vi "Self-Test.vi"(7 "Address":u16, 8 "Error In":errorcluster, 11 "VISA Resource in":refnum<visa-resource-name>) -> (0 "Error Out":errorcluster, 1 "Self-Test Result Message":string, 2 "Self-Test Result Code":i32, 3 "VISA Resource out":refnum<visa-resource-name>)   [LabVIEW 2014, in "KIT QV.lvlib"]
doc: "Runs the instrument's self-test routine and returns the test results."
uses:
  KIT QV.lvlib
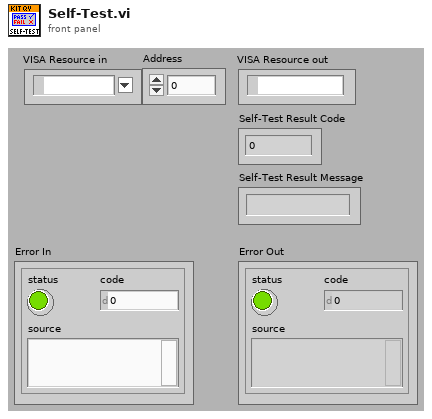
[diagram p1: front panel]
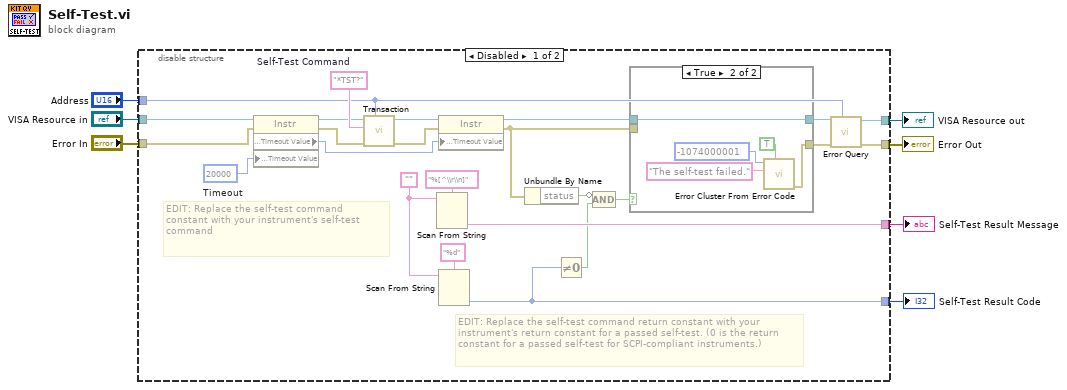
[diagram p0: block diagram]
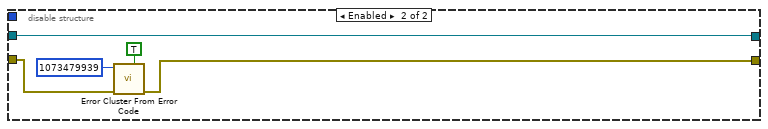
[diagram p3: hidden frame]
diagram:
  n1 = disable-structure shown="Disabled" {
    disable-tunnel: "VISA Resource in" -> [w29 w40]
    disable-tunnel: "Error In" -> [w28 w41]
    disable-tunnel: [w27 w40] -> w5
    disable-tunnel: [w26 w39] -> w4
    disable-tunnel: [w25 _] -> w3
    disable-tunnel: [w15 _] -> w2
    disable-tunnel: "Address" -> [w8 _]
    frame Disabled {
      w9 = ""
      w24 = u32 20000  # Timeout
      w14 = "*TST?"  # Self-Test Command
      # "EDIT: Replace the self-test command return constant with your instrument's return constant for a passed self-test. (0 is the return constant for a passed self-test for SCPI-compliant instruments.)"
      # "EDIT: Replace the self-test command constant with your instrument's self-test command"
      n2 = property class="Instr"(reference=w29, error in=w28, "General Settings:Timeout Value"=w24) -> (reference out=w13:refnum<visa-resource-name>, error out=w12:errorcluster, "General Settings:Timeout Value"=w23:u32)
      n3 = call "Transaction.vi"("Address"=w8, "error in (no error)"=w12, "Command"=w14, "VISA Resource in"=w13) -> ("error out"=w10:errorcluster, "VISA Resource out"=w11:refnum<visa-resource-name>)  [unwired: 5 in, 1 out]
      n4 = Scan From String(format string="%[^\\r\\n]" ("Format String"), input string=w9) -> (output 1=w25:string)  [unwired: 3 in, 3 out]
      n5 = property class="Instr"(reference=w11, error in=w10, "General Settings:Timeout Value"=w23) -> (reference out=w22:refnum<visa-resource-name>, error out=w21:errorcluster)
      n6 = Scan From String(format string="%d", input string=w9) -> (output 1=w15:i32)  [unwired: 3 in, 3 out]
      n7 = Unbundle By Name(w21) -> ("status"=w17:bool)
      n8 = Not Equal To 0?(x=w15) -> (x != 0?=w18:bool)
      n9 = Compound Arithmetic op=AND(invert w17, w18) -> (w16:bool)
      n10 = case shown="True" w16 {
        tunnel: w22 -> [w33 w38]
        tunnel: w21 -> [w32 _]
        tunnel: [w32 w34] -> w20
        tunnel: [w33 w38] -> w19
        frame False {
        }
        frame True {
          n11 = call <vilib>:"Error Cluster From Error Code.vi"("show call chain? (False)"=TRUE, "error message (\"\")"="The self-test failed." ("Source (VI Name)"), "error code (0)"=-1074000001 ("Code")) -> ("error out"=w34:errorcluster)  [unwired: 6 in]
        }
      }
      n12 = call "Error Query.vi"("Address"=w8, "Error in"=w20, "VISA Resource in"=w19) -> ("Error Out"=w26:errorcluster, "VISA Resource in"=w27:refnum<visa-resource-name>)  [unwired: 5 in, 2 out]
    }
    frame Enabled {
      n13 = call <vilib>:"Error Cluster From Error Code.vi"("is warning? (False)"=TRUE, "error in (no error)"=w41, "error code (0)"=1073479939) -> ("error out"=w39:errorcluster)  [unwired: 6 in]
    }
  }
  "Self-Test Result Message" <- w3
  "Self-Test Result Code" <- w2
  "VISA Resource out" <- w5
  "Error Out" <- w4
